vi "Solve Linear Equations (EXT).vi"(6 "Tolerance":dbl=0.001 format="%#_13g", 10 "b":ext[](array[numeric]), 11 "A":ext[][](array[numeric])) -> (2 "Out of Tolerance?":bool, 3 "X":ext[](array[numeric]))   [LabVIEW 2025, in "AOC.lvlib"]
uses:
  AOC.lvlib
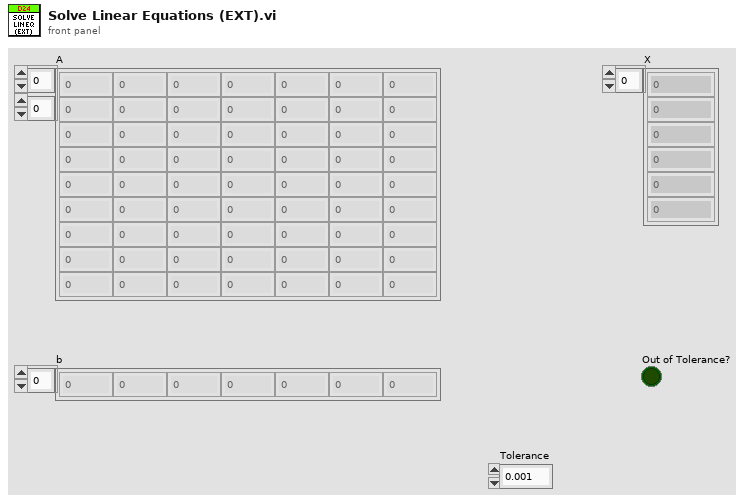
[diagram p1: front panel]
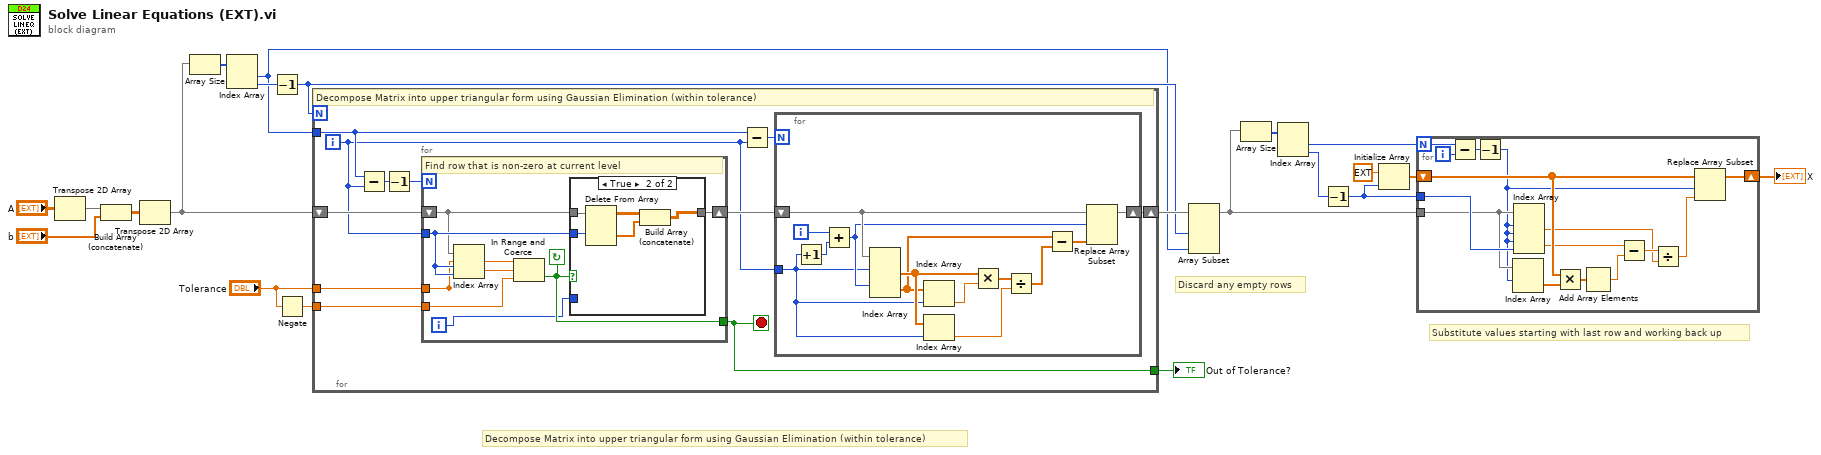
[diagram p0: block diagram]
diagram:
  # "Discard any empty rows"
  # "Substitute values starting with last row and working back up"
  # "Decompose Matrix into upper triangular form using Gaussian Elimination (within tolerance)"
  n1 = Transpose 2D Array(2D array="A") -> (transposed array=w6:ext[][])
  n2 = Build Array (concatenate)(w6, "b") -> (w5:ext[][])
  n3 = Transpose 2D Array(2D array=w5) -> (transposed array=w4:ext[][])
  n4 = Array Size(array=w4) -> (size(s)=w21:i32[])
  n5 = Index Array(array=w21) -> (element #1=w10:i32, element #2=w20:i32)  [unwired: 2 in]
  n6 = Decrement(x=w20) -> (x-1=w11:i32)
  n7 = Negate(x="Tolerance") -> (-x=w3:dbl)
  n8 = for {
    N: w11 -> [_]
    tunnel: w10 -> [w26]
    shift-right: [w32] -> w19
    shift-left: w4 -> [w30]
    tunnel: "Tolerance" -> [w28]
    tunnel: w3 -> [w27]
    tunnel: [w22] -> w1
    i -> [w25]
    stop <- w22 stop-if-true
    # "Decompose Matrix into upper triangular form using Gaussian Elimination (within tolerance)"
    n9 = Subtract(x=w26, y=w25) -> (x-y=w24:i32)
    n10 = Decrement(x=w24) -> (x-1=w23:i32)
    n11 = for {
      N: w23 -> [_]
      tunnel: w25 -> [w40]
      shift-right: [w38] -> w29
      shift-left: w30 -> [w39]
      tunnel: w28 -> [w36]
      tunnel: [w36] -> _
      tunnel: w27 -> [w35]
      tunnel: [w34] -> w22
      i -> [w33]
      stop <- w34 continue-if-true
      # "Find row that is non-zero at current level"
      n12 = Index Array(array=w39, index (row)=w40, index (col)=w40) -> (element=w37:ext)
      n13 = In Range and Coerce(upper limit=w36, x=w37, lower limit=w35) -> (In Range?=w34:bool)  [unwired: 1 out]
      n14 = case shown="True" w34 {
        tunnel: w40 -> [_ w45]
        tunnel: w39 -> [w41 w46]
        tunnel: [w41 w42] -> w38
        tunnel: w33 -> [_ _]
        frame False {
        }
        frame True {
          n15 = Delete From Array(array=w46, index (row)=w45) -> (deleted portion=w43:ext[], array with subset deleted=w44:ext[][])  [unwired: 2 in]
          n16 = Build Array (concatenate)(w44, w43) -> (w42:ext[][])
        }
      }
    }
    n17 = Subtract(x=w26, y=w25) -> (x-y=w31:i32)
    n18 = for {
      N: w31 -> [_]
      tunnel: w25 -> [w50]
      shift-right: [w55] -> w32
      shift-left: w29 -> [w56]
      i -> [w52]
      n19 = Increment(x=w50) -> (x+1=w51:i32)
      n20 = Add(x=w52, y=w51) -> (x+y=w53:i32)
      n21 = Index Array(array=w56, index (row) #1=w50, index (row) #2=w53) -> (element #1=w58:ext[], element #2=w57:ext[])  [unwired: 2 in]
      n22 = Index Array(array=w57, index=w50) -> (element=w49:ext)
      n23 = Index Array(array=w58, index=w50) -> (element=w59:ext)
      n24 = Multiply(x=w58, y=w49) -> (x*y=w48:ext[])
      n25 = Divide(x=w48, y=w59) -> (x/y=w47:ext[])
      n26 = Subtract(x=w57, y=w47) -> (x-y=w54:ext[])
      n27 = Replace Array Subset(array=w56, new element=w54, index (row)=w53) -> (w55:ext[][])  [unwired: 1 in]
    }
  }
  "Out of Tolerance?" <- w1
  n28 = Array Subset(array=w19, length (row)=w11, length (col)=w10) -> (w12:ext[][])  [unwired: 2 in]
  n29 = Array Size(array=w12) -> (size(s)=w18:i32[])
  n30 = Index Array(array=w18) -> (element #1=w17:i32, element #2=w9:i32)  [unwired: 2 in]
  n31 = Decrement(x=w9) -> (x-1=w8:i32)
  n32 = Initialize Array(ext 0.0, w8) -> (w14:ext[])
  n33 = for {
    N: w17 -> [w74]
    tunnel: w12 -> [w68]
    tunnel: w8 -> [w72]
    shift-right: [w71] -> w16
    shift-left: w14 -> [w70]
    i -> [w73]
    n34 = Subtract(x=w74, y=w73) -> (x-y=w65:i32)
    n35 = Decrement(x=w65) -> (x-1=w64:i32)
    n36 = Index Array(array=w68, index (row)=w64) -> (element=w67:ext[])  [unwired: 1 in]
    n37 = Index Array(array=w68, index (row) #1=w64, index (col) #1=w64, index (row) #2=w64, index (col) #2=w72) -> (element #1=w60:ext, element #2=w62:ext)
    n38 = Multiply(x=w70, y=w67) -> (x*y=w69:ext[])
    n39 = Add Array Elements(numeric array=w69) -> (sum=w61:ext)
    n40 = Subtract(x=w62, y=w61) -> (x-y=w63:ext)
    n41 = Divide(x=w63, y=w60) -> (x/y=w66:ext)
    n42 = Replace Array Subset(array=w70, new element=w66, index=w64) -> (w71:ext[])
  }
  "X" <- w16
